vi "Voorbeeld_State_Machine_01_sequence.vi"() -> ()   [LabVIEW 2019]
panel:
  out "String":string
  in  "stop":bool
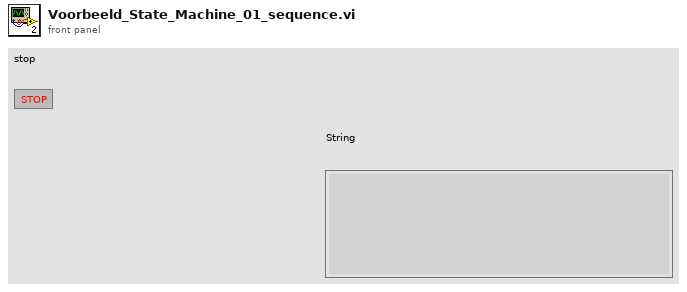
[diagram p1: front panel]
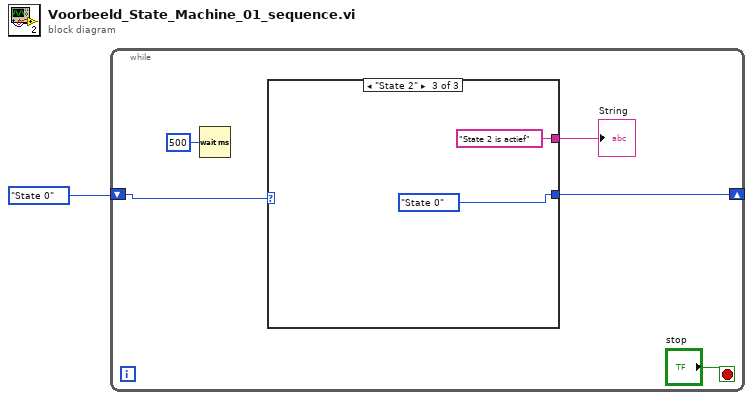
[diagram p0: block diagram]
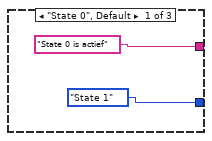
[diagram p2: hidden frame]
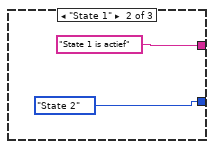
[diagram p3: hidden frame]
diagram:
  n1 = while {
    shift-right: [w3] -> _
    shift-left: enum16{"State 0", "State 1", "State 2"}."State 0" -> [w5]
    stop <- "stop" stop-if-true
    n2 = Wait (ms)(milliseconds to wait=u32 500) -> ()  [unwired: 1 out]
    n3 = case shown="\"State 2\"" w5 {
      tunnel: ["State 0 is actief" ("String") "State 1 is actief" ("String") "State 2 is actief" ("String")] -> w4
      tunnel: [enum16{"State 0", "State 1", "State 2"}."State 1" enum16{"State 0", "State 1", "State 2"}."State 2" enum16{"State 0", "State 1", "State 2"}."State 0"] -> w3
      frame "State 0", Default {
      }
      frame "State 1" {
      }
      frame "State 2" {
      }
    }
    "String" <- w4
  }
